vi "DisplayManager.vi"(2 "isColorActive":bool[](array[boolean])=[TRUE, TRUE, TRUE, TRUE, TRUE], 3 "Color Lists":T3, 4 "Display type":u8(ring) items=["Outlined", "Filled", ""], 5 "RTGDataPack":T1) -> (1 "Output Image":T2)   [LabVIEW 2014]
doc: "Umozliwia wyświetlanie obrysów ROI lub wypełnionych ROI. ROI są wyszczególnione w tablicy Color List. Obsługiwane jest 6 grup które mogą być oznaczane różnymi kolorami. Pierwsza grupa zawsze jest wyświetlana, pozostałe pięć może być wyświetlane opcjonalnie"
uses:
  <vilib>/vision/Image Controls.llb/IMAQ Image.ctl
  DataTypes/DataTypes.llb/Indexes.ctl
  DataTypes/DataTypes.llb/RTG.ctl
  <vilib>/vision/NI_Vision_Development_Module.lvlib
panel:
  out "over":T2(plugin-control)
  out "label":T2(plugin-control)
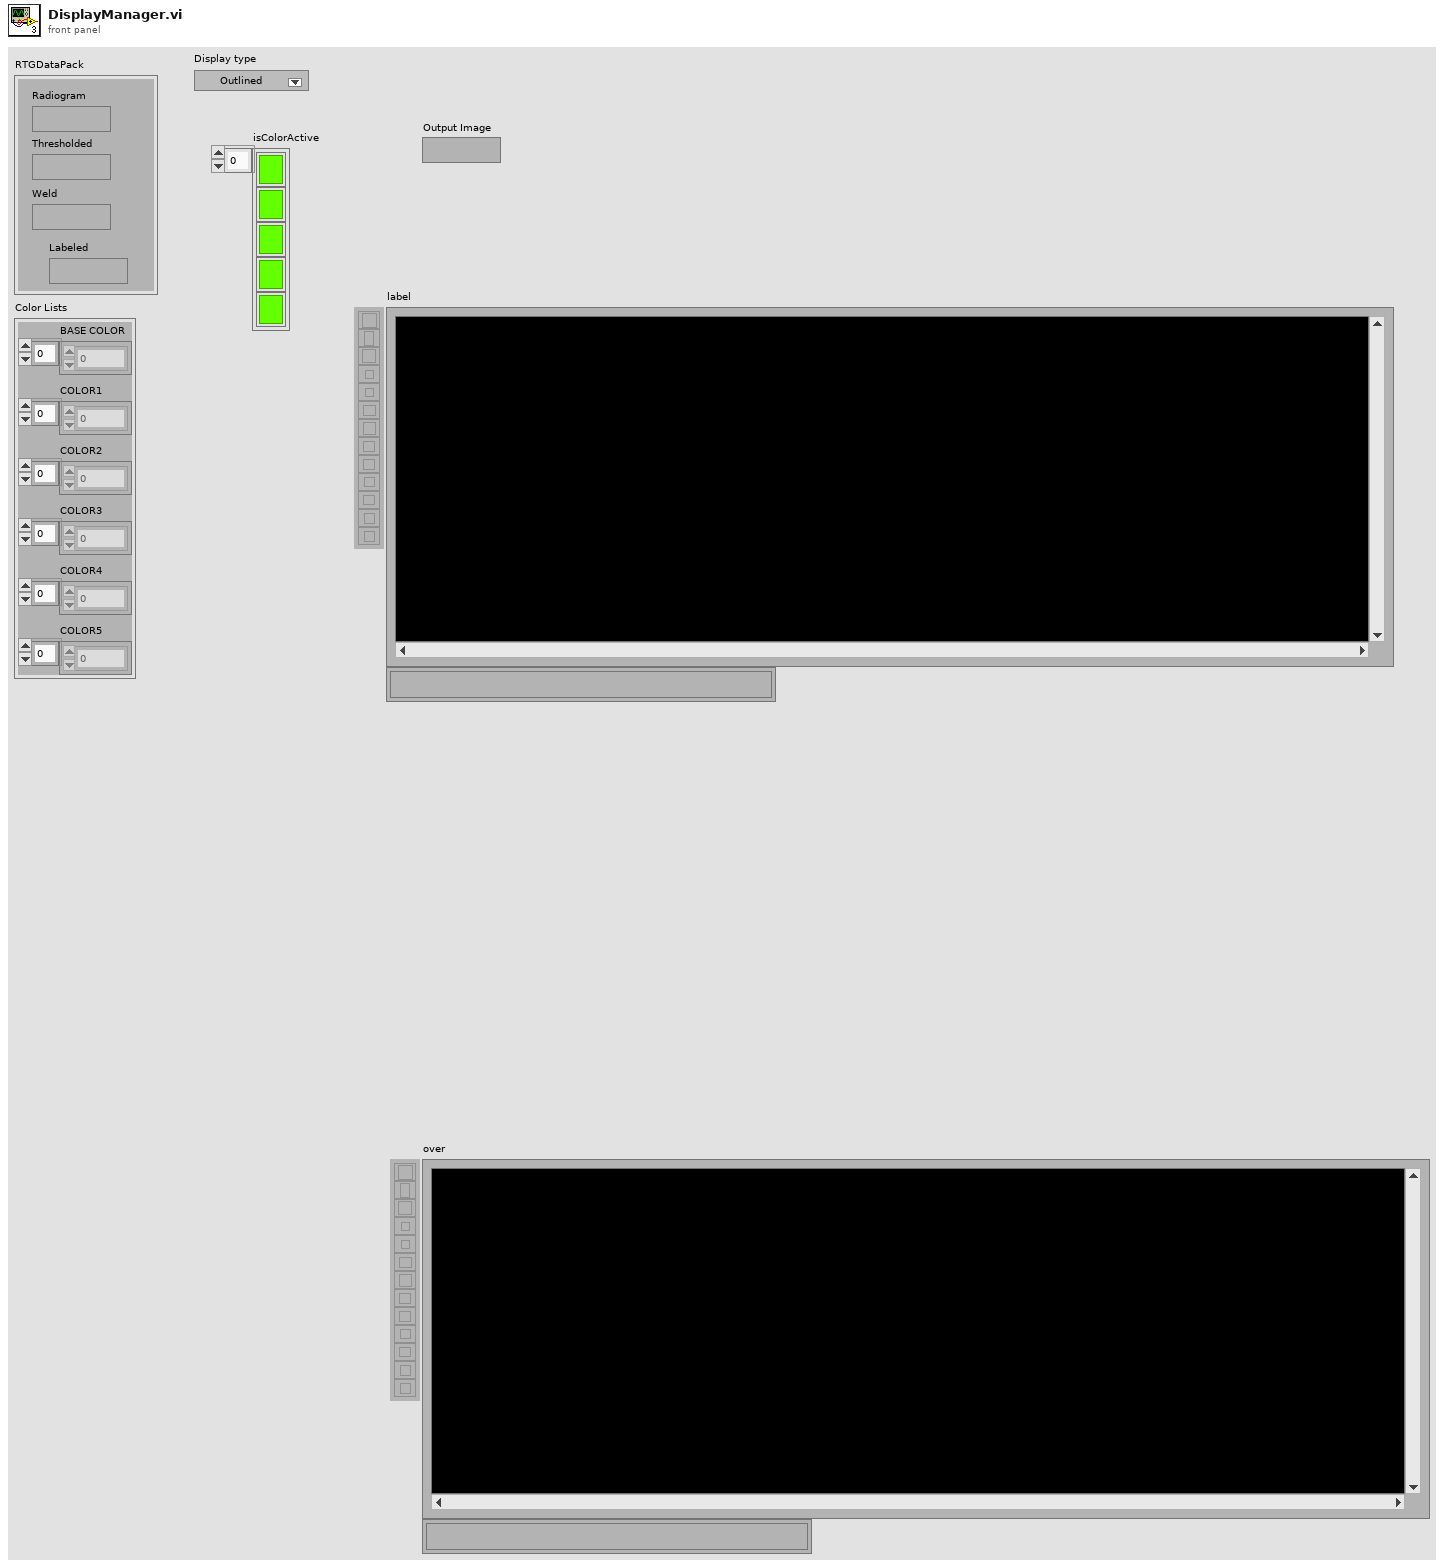
[diagram p1: front panel]
types:
  T1 = typedef "RTG.ctl" = cluster{"Radiogram":T2, "Thresholded":T2, "Weld":T2, "Labeled":T2}
  T2 = typedef "IMAQ Image.ctl" = refnum<image>
  T3 = typedef "Indexes.ctl" = cluster{"BASE COLOR":dbl[], "COLOR1":dbl[], "COLOR2":dbl[], "COLOR3":dbl[], "COLOR4":dbl[], "COLOR5":dbl[]}
  T4 = typedef "Image Type" = u32
  T5 = typedef "ROI Descriptor" = cluster{"Global Rectangle":i32[], "Contours":cluster{"ID":enum32{"External", "Internal"}, "Type":u32, "Coordinates":i32[]}[]}
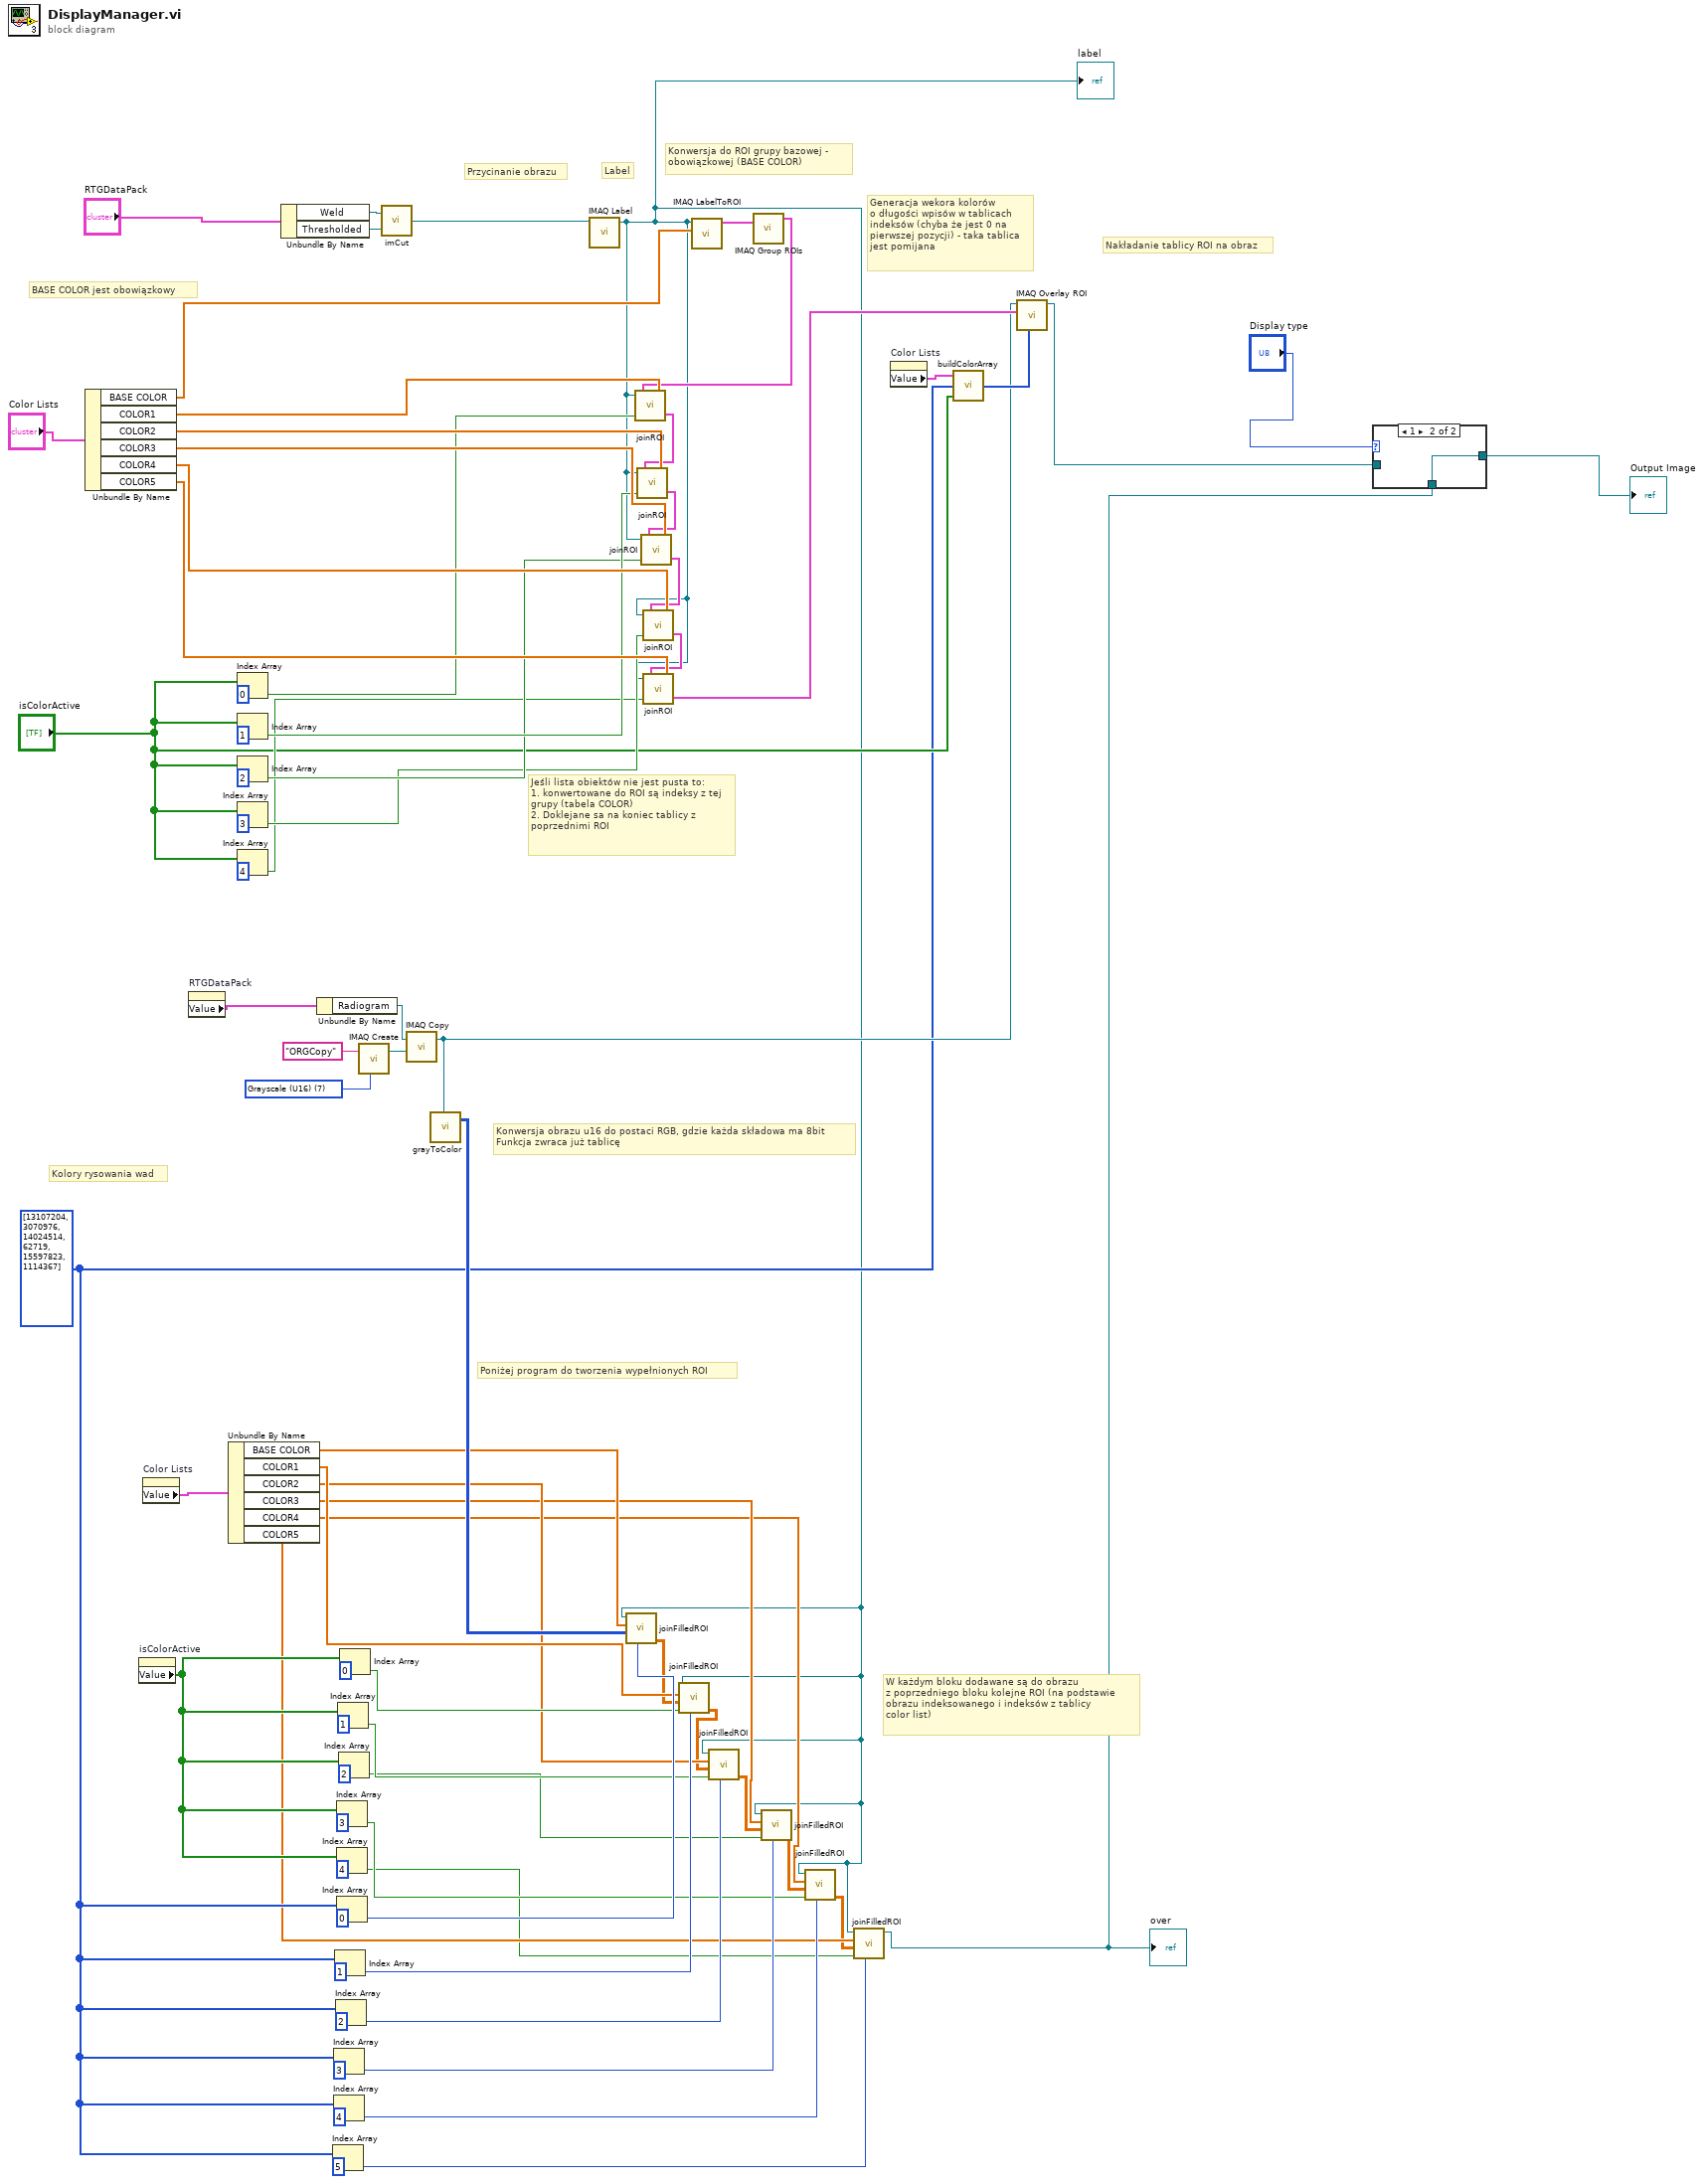
[diagram p0: block diagram]
diagram:
  w26 = u32[] [13107204, 3070976, 14024514, 62719, 15597823, 1114367] ("Colors")
  w78 = T4 7 items=["Grayscale (U8)", "Grayscale (I16)", "Grayscale (SGL)", "Complex (CSG)", "RGB (U32)", "HSL (U32)", "RGB (U64)", "Grayscale (U16)"] ("Image Type")
  # "W każdym bloku dodawane są do obrazu\nz poprzedniego bloku kolejne ROI (na podstawie\nobrazu indeksowanego i indeksów z tablicy \ncolor list)"
  # "Konwersja obrazu u16 do postaci RGB, gdzie każda składowa ma 8bit\nFunkcja zwraca już tablicę"
  # "Poniżej program do tworzenia wypełnionych ROI"
  # "Kolory rysowania wad"
  # "Jeśli lista obiektów nie jest pusta to:\n1. konwertowane do ROI są indeksy z tej grupy (tabela COLOR)\n2. Doklejane sa na koniec tablicy z poprzednimi ROI"
  # "Nakładanie tablicy ROI na obraz"
  # "Generacja wekora kolorów\no długości wpisów w tablicach\nindeksów (chyba że jest 0 na \npierwszej pozycji) - taka tablica\njest pomijana"
  # "BASE COLOR jest obowiązkowy"
  # "Konwersja do ROI grupy bazowej - \nobowiązkowej (BASE COLOR)"
  # "Label"
  # "Przycinanie obrazu"
  n1 = Unbundle By Name("Color Lists") -> ("BASE COLOR"=w43:dbl[], "COLOR1"=w65:dbl[], "COLOR2"=w63:dbl[], "COLOR3"=w62:dbl[], "COLOR4"=w61:dbl[], "COLOR5"=w60:dbl[])
  n2 = property on="isColorActive" class="Arr (strict)"() -> ("Value"=w34:bool[])  [unwired: 2 in, 2 out]
  n3 = property on="Color Lists" class="Clust (strict)"() -> ("Value"=w40:T3)  [unwired: 2 in, 2 out]
  n4 = property on="RTGDataPack" class="Clust (strict)"() -> ("Value"=w1:T1)  [unwired: 2 in, 2 out]
  n5 = Unbundle By Name(w40) -> ("BASE COLOR"=w28:dbl[], "COLOR1"=w24:dbl[], "COLOR2"=w20:dbl[], "COLOR3"=w16:dbl[], "COLOR4"=w12:dbl[], "COLOR5"=w7:dbl[])
  n6 = Index Array(array="isColorActive", index=0) -> (element=w49:bool)
  n7 = Index Array(array="isColorActive", index=1) -> (element=w48:bool)
  n8 = Index Array(array="isColorActive", index=2) -> (element=w47:bool)
  n9 = Index Array(array="isColorActive", index=3) -> (element=w46:bool)
  n10 = Index Array(array="isColorActive", index=4) -> (element=w45:bool)
  n11 = Unbundle By Name("RTGDataPack") -> ("Weld"=w71:T2, "Thresholded"=w70:T2)
  n12 = Unbundle By Name(w1) -> ("Radiogram"=w67:T2)
  n13 = Index Array(array=w26, index=5) -> (element=w4:u32)
  n14 = Index Array(array=w26, index=3) -> (element=w13:u32)
  n15 = Index Array(array=w26, index=4) -> (element=w9:u32)
  n16 = Index Array(array=w26, index=1) -> (element=w21:u32)
  n17 = Index Array(array=w26, index=2) -> (element=w17:u32)
  n18 = Index Array(array=w34, index=3) -> (element=w10:bool)
  n19 = Index Array(array=w34, index=4) -> (element=w5:bool)
  n20 = Index Array(array=w26, index=0) -> (element=w25:u32)
  n21 = Index Array(array=w34, index=1) -> (element=w18:bool)
  n22 = Index Array(array=w34, index=2) -> (element=w14:bool)
  n23 = Index Array(array=w34, index=0) -> (element=w22:bool)
  n24 = call "IMAQ Create"("Image Name"="ORGCopy", "Image Type"=w78) -> ("New Image"=w76:T2)  [unwired: 3 in, 1 out]
  n25 = call "imCut.vi"("Image Src"=w70, "Image Mask"=w71) -> ("Image Out"=w75:T2)
  n26 = call "IMAQ Copy"("Image Dst"=w76, "Image Src"=w67) -> ("Image Dst Out"=w42:T2)  [unwired: 4 in, 1 out]
  n27 = call "grayToColor.vi"("U16 Image"=w42) -> ("RGB array"=w41:u32[][])  [unwired: 1 in, 1 out]
  n28 = call "IMAQ Label"("Image Src"=w75) -> ("Image Dst Out"=w8:T2)  [unwired: 3 in, 2 out]
  "label" <- w8
  n29 = call "joinFilledROI.vi"("Color"=w25, "Image Array"=w41, "COLOR Array"=w28, "Labeled Image"=w8) -> ("Image Out Array"=w23:dbl[][])  [unwired: 6 in, 1 out]
  n30 = call "joinFilledROI.vi"("Color"=w21, "isActive"=w22, "Image Array"=w23, "COLOR Array"=w24, "Labeled Image"=w8) -> ("Image Out Array"=w19:dbl[][])  [unwired: 5 in, 1 out]
  n31 = call "IMAQ LabelToROI"("Labels In"=w43, "Image"=w8) -> ("ROIs"=w79:T5[])  [unwired: 6 in, 3 out]
  n32 = call "joinFilledROI.vi"("Color"=w17, "isActive"=w18, "Image Array"=w19, "COLOR Array"=w20, "Labeled Image"=w8) -> ("Image Out Array"=w15:dbl[][])  [unwired: 5 in, 1 out]
  n33 = call "IMAQ Group ROIs"("ROI Descriptors"=w79) -> ("ROI Descriptor out"=w64:T5)  [unwired: 3 in, 1 out]
  n34 = call "joinROI.vi"("COLOR Array"=w65, "isActive"=w49, "ROI Descriptor in"=w64, "Labeled image"=w8) -> ("ROI Descriptor out"=w59:T5)
  n35 = call "joinROI.vi"("COLOR Array"=w63, "isActive"=w48, "ROI Descriptor in"=w59, "Labeled image"=w8) -> ("ROI Descriptor out"=w58:T5)
  n36 = call "joinROI.vi"("COLOR Array"=w62, "isActive"=w47, "ROI Descriptor in"=w58, "Labeled image"=w8) -> ("ROI Descriptor out"=w57:T5)
  n37 = call "joinROI.vi"("COLOR Array"=w61, "isActive"=w46, "ROI Descriptor in"=w57, "Labeled image"=w8) -> ("ROI Descriptor out"=w56:T5)
  n38 = call "joinROI.vi"("COLOR Array"=w60, "isActive"=w45, "ROI Descriptor in"=w56, "Labeled image"=w8) -> ("ROI Descriptor out"=w55:T5)
  n39 = call "joinFilledROI.vi"("Color"=w13, "isActive"=w14, "Image Array"=w15, "COLOR Array"=w16, "Labeled Image"=w8) -> ("Image Out Array"=w11:dbl[][])  [unwired: 5 in, 1 out]
  n40 = call "joinFilledROI.vi"("Color"=w9, "isActive"=w10, "Image Array"=w11, "COLOR Array"=w12, "Labeled Image"=w8) -> ("Image Out Array"=w6:dbl[][])  [unwired: 5 in, 1 out]
  n41 = call "joinFilledROI.vi"("Color"=w4, "isActive"=w5, "Image Array"=w6, "COLOR Array"=w7, "Labeled Image"=w8) -> ("Image out"=w3:T2)  [unwired: 5 in, 1 out]
  "over" <- w3
  n42 = property on="Color Lists" class="Clust (strict)"() -> ("Value"=w66:T3)  [unwired: 2 in, 2 out]
  n43 = call "buildColorArray.vi"("isColorActive"="isColorActive", "Colors"=w26, "Color Lists"=w66) -> ("output array"=w69:u32[])
  n44 = call "IMAQ Overlay ROI"("Colors (Green)"=w69, "ROI Descriptor"=w55, "Image"=w42) -> ("Image Out"=w74:T2)  [unwired: 7 in, 1 out]
  n45 = case shown="1" "Display type" {
    tunnel: w74 -> [w80 _]
    tunnel: [w80 w81] -> w73
    tunnel: w3 -> [_ w81]
    frame 0, Default {
    }
    frame 1 {
    }
  }
  "Output Image" <- w73
